vi "Create chapter and section.vi"(0 "PDF Report IN":refnum<class "PDF Report Class.lvclass">, 2 "TriggerNewPage":bool, 5 "Chapter or section IN":T1, 7 "Paragragh":refnum<k24>, 11 "error in (no error)":errorcluster, 13 "BookmarkOpen":bool=TRUE) -> (4 "PDF Report OUT":refnum<class "PDF Report Class.lvclass">, 8 "Chapter":refnum<k24>, 10 "Section":refnum<k24>, 15 "error out":errorcluster)   [LabVIEW 2019]
doc: "Version 1.1\nDeveloped by Jean-Marc Simard\nCopyright © 2012, Exaprom Inc.\nAll rights reserved.\nLicense: BSD\n\nWith iTextSharp 4.1.6 (http://itextsharp.sourceforge.net)\nunder Mozilla Public License Version 1.1\n(http://www.mozilla.org/MPL/MPL-1.1.html)"
uses:
  <userlib>/Exaprom PDF/LV Class/PDF Report Class/PDF Report Class.lvclass
  <userlib>/Exaprom PDF/Controls/Chapter Controls/Chapter.ctl
  C:/Program Files/National Instruments/LabVIEW 2019/user.lib/Exaprom PDF/DLL/itextsharp.dll
  DLL/itextsharp.dll
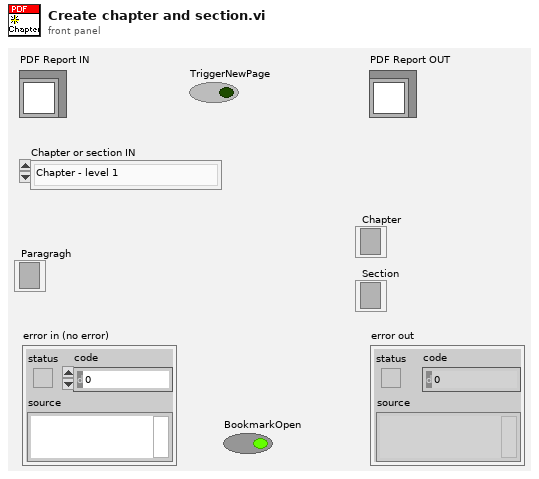
[diagram p1: front panel]
types:
  T1 = typedef "Chapter.ctl" = enum16{"Chapter - level 1", "Chapter - level 2", "Chapter - level 3", "Chapter - level 4"}
  T2 = cluster{"ChapterAutoNumber":refnum<k24>, "Section [ ]":refnum<k24>[]}
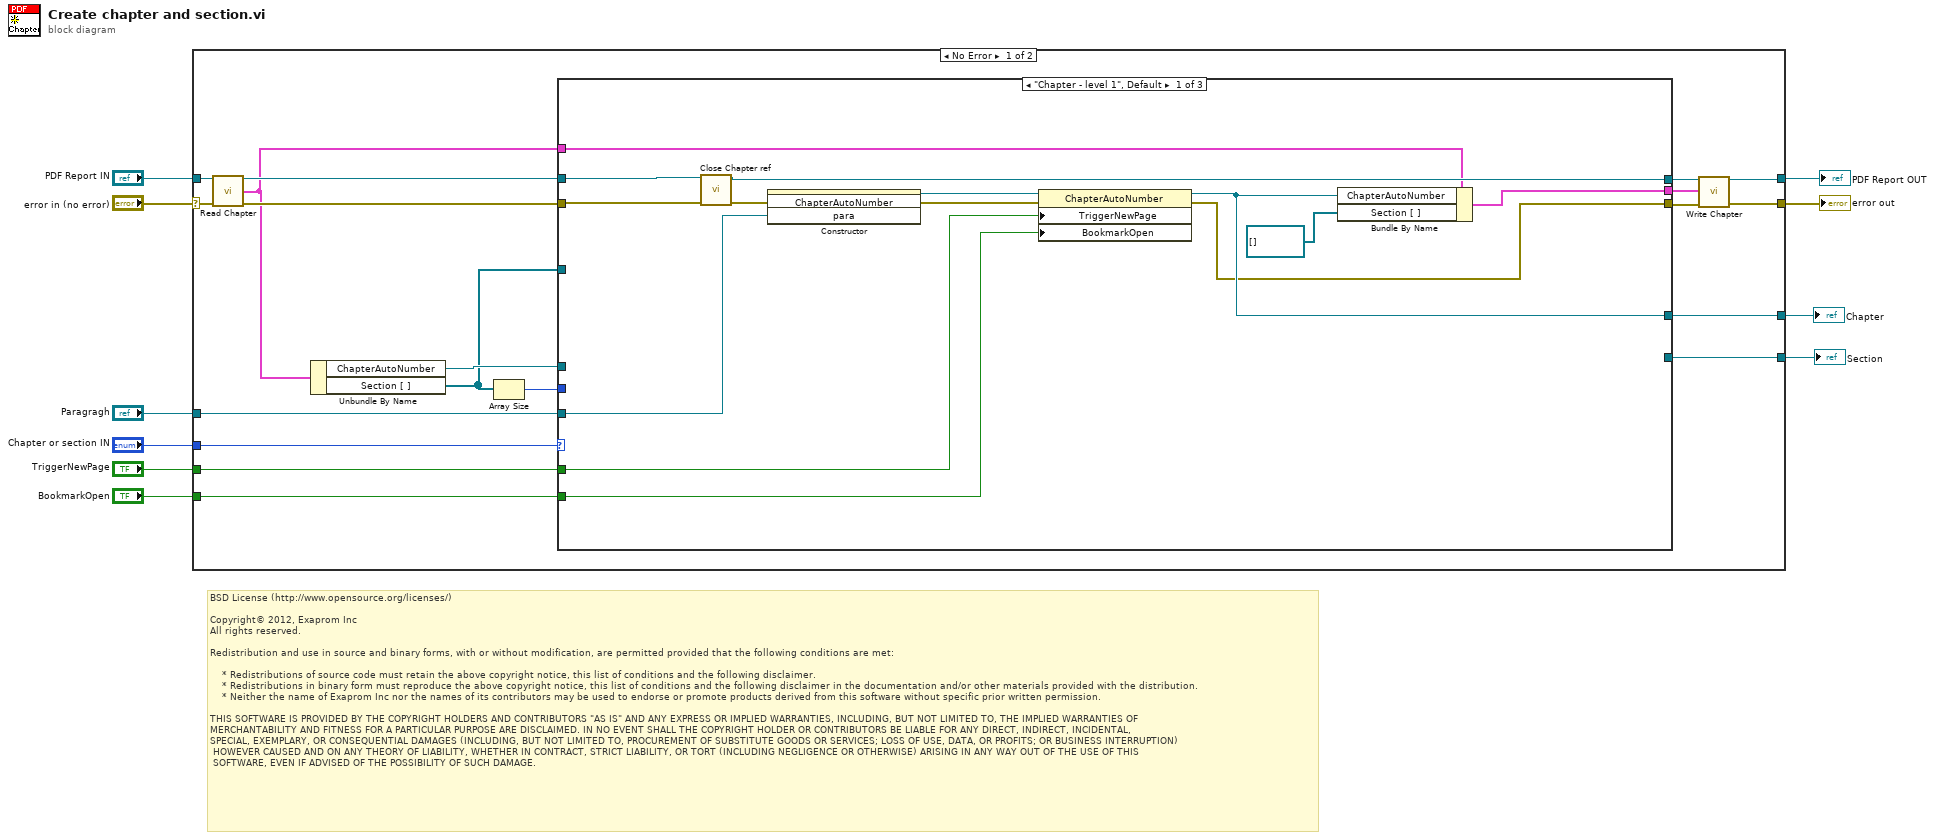
[diagram p0: block diagram]
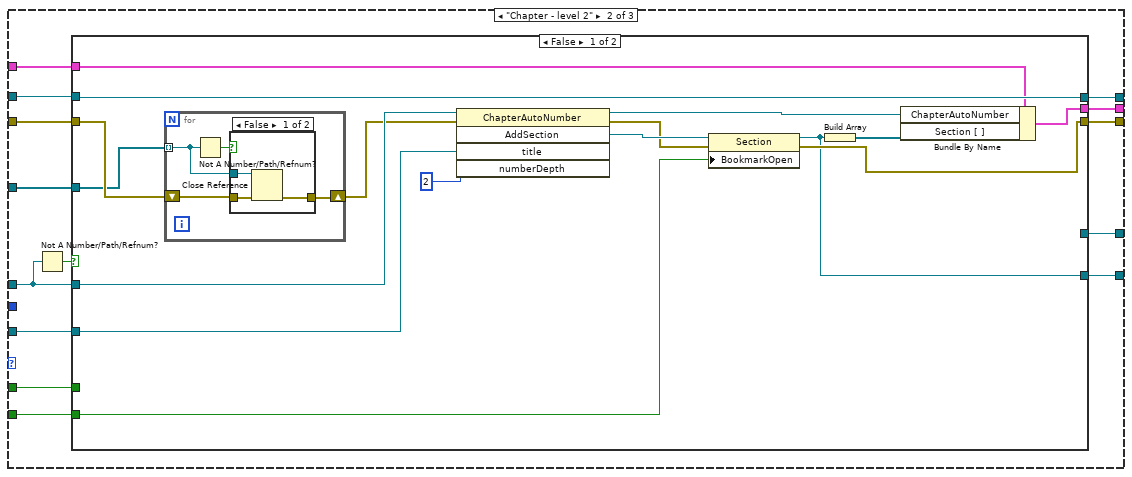
[diagram p2: hidden frame]
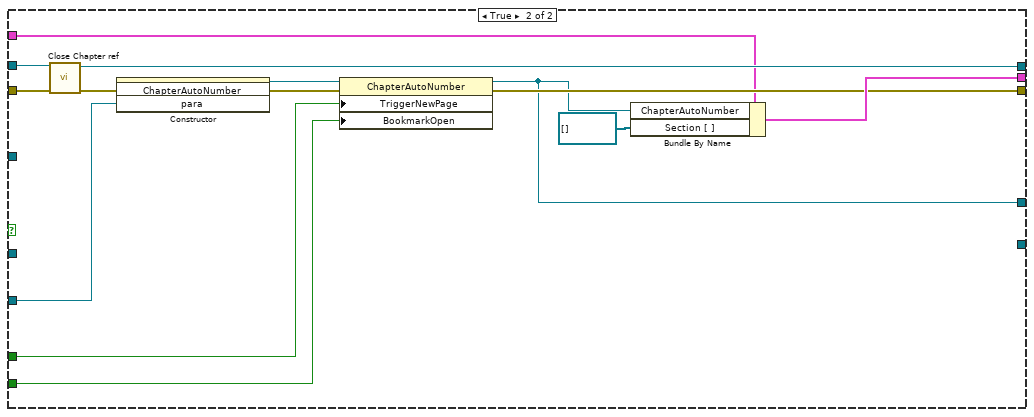
[diagram p4: hidden frame]
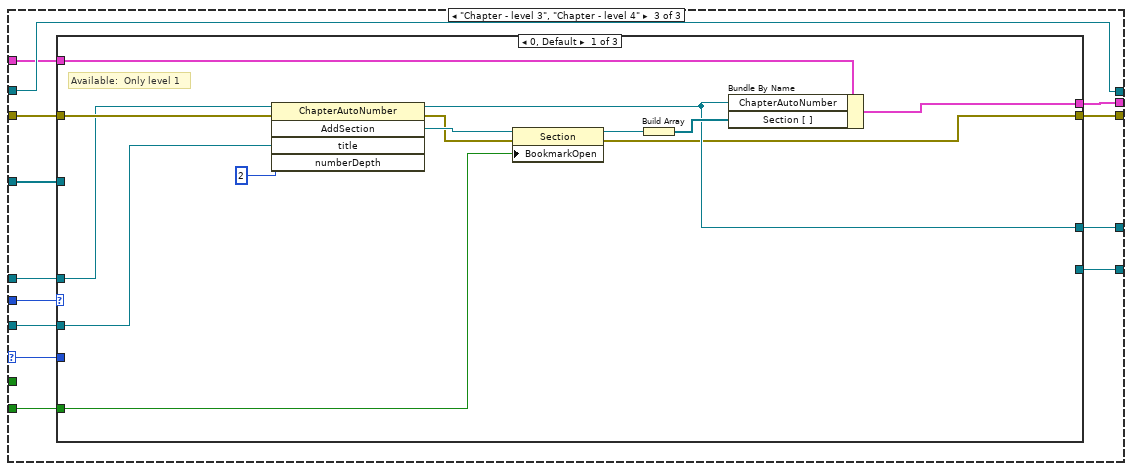
[diagram p5: hidden frame]
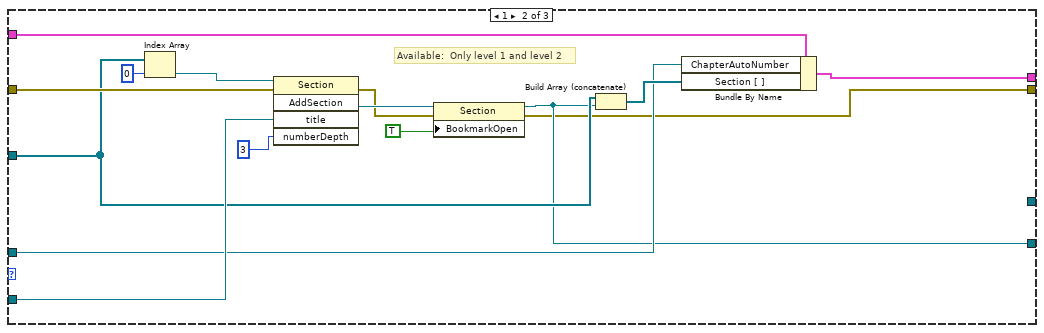
[diagram p6: hidden frame]
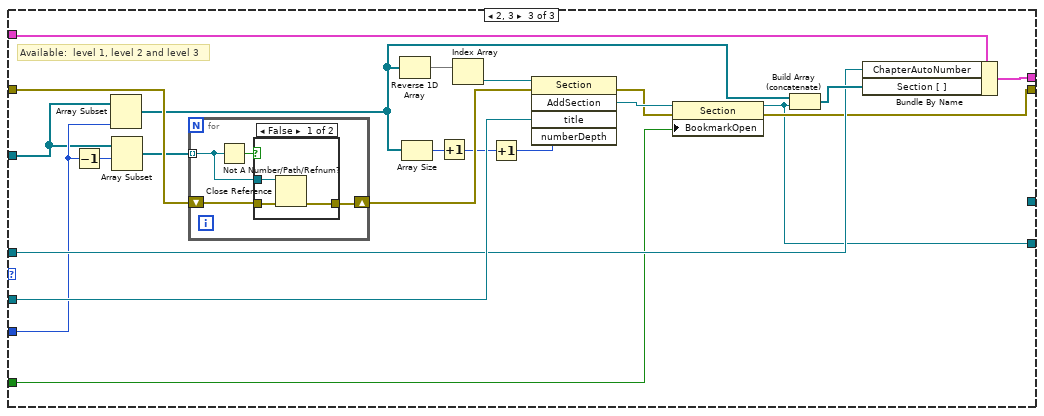
[diagram p7: hidden frame]
diagram:
  # "BSD License (http://www.opensource.org/licenses/)\n\nCopyright© 2012, Exaprom Inc\nAll rights reserved.\n\nRedistribution and use in source and binary forms, with or without modification, are permitted provided that the following conditions are met:\n\n    * Redistributions of source code must retain the above copyright notice, this list of conditions and the following disclaimer.\n    * Redistributions in binary form must reproduce the above copyright notice, this list of conditions and the following disclaimer in the documentation and/or other materials provided with the distribution.\n    * Neither the name of Exaprom Inc nor the names of its contributors may be used to endorse or promote products derived from this software without specific prior written permission.\n\nTHIS SOFTWARE IS PROVIDED BY THE COPYRIGHT HOLDERS AND CONTRIBUTORS \"AS IS\" AND ANY EXPRESS OR IMPLIED WARRANTIES, INCLUDING, BUT NOT LIMITED TO, THE IMPLIED WARRANTIES OF \nMERCHANTABILITY AND FITNESS FOR A PARTICULAR PURPOSE ARE DISCLAIMED. IN NO EVENT SHALL THE COPYRIGHT HOLDER OR CONTRIBUTORS BE LIABLE FOR ANY DIRECT, INDIRECT, INCIDENTAL,\nSPECIAL, EXEMPLARY, OR CONSEQUENTIAL DAMAGES (INCLUDING, BUT NOT LIMITED TO, PROCUREMENT OF SUBSTITUTE GOODS OR SERVICES; LOSS OF USE, DATA, OR PROFITS; OR BUSINESS INTERRUPTION)\n HOWEVER CAUSED AND ON ANY THEORY OF LIABILITY, WHETHER IN CONTRACT, STRICT LIABILITY, OR TORT (INCLUDING NEGLIGENCE OR OTHERWISE) ARISING IN ANY WAY OUT OF THE USE OF THIS\n SOFTWARE, EVEN IF ADVISED OF THE POSSIBILITY OF SUCH DAMAGE."
  n1 = case shown="No Error" "error in (no error)" {
    selector: "error in (no error)" -> [w28 w168]
    tunnel: "PDF Report IN" -> [w29 w167]
    tunnel: [w18 w167] -> w9
    tunnel: [w21 w168] -> w8
    tunnel: "Chapter or section IN" -> [w27 _]
    tunnel: "Paragragh" -> [w23 _]
    tunnel: [w15 _] -> w4
    tunnel: [w14 _] -> w3
    tunnel: "TriggerNewPage" -> [w13 _]
    tunnel: "BookmarkOpen" -> [w11 _]
    frame No Error {
      n2 = call-dynamic "Read Chapter.vi"("PDF Report Class in"=w29, "error in (no error)"=w28) -> ("PDF Report Class out"=w17:refnum<class "PDF Report Class.lvclass">, "Chapter ref"=w12:T2, "error out"=w26:errorcluster)  [unwired: 11 in]
      n3 = Unbundle By Name(w12) -> ("ChapterAutoNumber"=w24:refnum<k24>, "Section [ ]"=w22:refnum<k24>[])
      n4 = Array Size(array=w22) -> (size(s)=w25:i32)
      n5 = case shown="\"Chapter - level 1\", Default" w27 {
        selector: w27 -> [_ _ w101]
        tunnel: w26 -> [w34 w56 w104]
        tunnel: w25 -> [_ _ w108]
        tunnel: w24 -> [_ w51 w103]
        tunnel: w23 -> [w36 w57 w102]
        tunnel: [w32 w53 w105] -> w20
        tunnel: w22 -> [_ w55 w107]
        tunnel: [w39 w54 w106] -> w19
        tunnel: w17 -> [w33 w50 w100]
        tunnel: [w41 w49 w100] -> w16
        tunnel: [w37 w48 w98] -> w15
        tunnel: [_ w47 w99] -> w14
        tunnel: w13 -> [w38 w46 _]
        tunnel: w12 -> [w35 w45 w97]
        tunnel: w11 -> [w31 w44 w96]
        frame "Chapter - level 1", Default {
          n6 = call <userlib>:"Close Chapter ref.vi"("PDF Report IN"=w33, "error in (no error)"=w34) -> ("PDF Report OUT"=w41:refnum<class "PDF Report Class.lvclass">, "error out"=w42:errorcluster)  [unwired: 12 in]
          n7 = constructor class="ChapterAutoNumber"(error in=w42, "para"=w36) -> (reference out=w30:refnum<k24>, error out=w43:errorcluster)  [unwired: 2 in, 2 out]
          n8 = property class="ChapterAutoNumber"(reference=w30, error in=w43, "TriggerNewPage"=w38, "BookmarkOpen"=w31) -> (reference out=w37:refnum<k24>, error out=w32:errorcluster)
          n9 = Bundle By Name(cluster=w35, "ChapterAutoNumber"=w37, "Section [ ]"=refnum<k24>[] []) -> (w39:T2)
        }
        frame "Chapter - level 2" {
          n10 = Not A Number/Path/Refnum?(number/path/refnum=w51) -> (NaN/Path/Refnum?=w52:bool)
          n11 = case shown="False" w52 {
            tunnel: w51 -> [w73 _]
            tunnel: w57 -> [w72 w86]
            tunnel: w56 -> [w68 w91]
            tunnel: w55 -> [w66 _]
            tunnel: [w65 w90] -> w54
            tunnel: [w62 w88] -> w53
            tunnel: w50 -> [w61 w89]
            tunnel: [w61 w87] -> w49
            tunnel: [_ w85] -> w48
            tunnel: [w60 _] -> w47
            tunnel: w46 -> [_ w83]
            tunnel: w45 -> [w59 w84]
            tunnel: w44 -> [w58 w82]
            frame False {
              n12 = for {
                shift-right: [w75] -> w67
                shift-left: w68 -> [w76]
                tunnel: w66 -> [w74] mode=indexing
                n13 = Not A Number/Path/Refnum?(number/path/refnum=w74) -> (NaN/Path/Refnum?=w77:bool)
                n14 = case shown="False" w77 {
                  tunnel: w74 -> [w80 _]
                  tunnel: w76 -> [w79 w81]
                  tunnel: [w78 w81] -> w75
                  frame False {
                    n15 = Close Reference(reference=w80, error in (no error)=w79) -> (error out=w78:errorcluster)
                  }
                  frame True {
                  }
                }
              }
              n16 = invoke class="ChapterAutoNumber" method="AddSection"(reference=w73, error in=w67, "title"=w72, "numberDepth"=2) -> (reference out=w69:refnum<k24>, error out=w63:errorcluster, "AddSection"=w64:refnum<k24>)  [unwired: 1 in, 2 out]
              n17 = property class="Section"(reference=w64, error in=w63, "BookmarkOpen"=w58) -> (reference out=w60:refnum<k24>, error out=w62:errorcluster)
              n18 = Build Array(w60) -> (w70:refnum<k24>[])
              n19 = Bundle By Name(cluster=w59, "ChapterAutoNumber"=w69, "Section [ ]"=w70) -> (w65:T2)
            }
            frame True {
              n20 = call <userlib>:"Close Chapter ref.vi"("PDF Report IN"=w89, "error in (no error)"=w91) -> ("PDF Report OUT"=w87:refnum<class "PDF Report Class.lvclass">, "error out"=w93:errorcluster)  [unwired: 12 in]
              n21 = constructor class="ChapterAutoNumber"(error in=w93, "para"=w86) -> (reference out=w94:refnum<k24>, error out=w95:errorcluster)  [unwired: 2 in, 2 out]
              n22 = property class="ChapterAutoNumber"(reference=w94, error in=w95, "TriggerNewPage"=w83, "BookmarkOpen"=w82) -> (reference out=w85:refnum<k24>, error out=w88:errorcluster)
              n23 = Bundle By Name(cluster=w84, "ChapterAutoNumber"=w85, "Section [ ]"=refnum<k24>[] []) -> (w90:T2)
            }
          }
        }
        frame "Chapter - level 3", "Chapter - level 4" {
          n24 = case shown="0, Default" w108 {
            tunnel: w107 -> [_ w128 w148]
            tunnel: [w112 w123 w142] -> w105
            tunnel: [w119 w134 w156] -> w106
            tunnel: w104 -> [w118 w133 w158]
            tunnel: w103 -> [w117 w129 w154]
            tunnel: w102 -> [w111 w132 w155]
            tunnel: w101 -> [_ _ w151]
            tunnel: [_ w124 w141] -> w99
            tunnel: [w116 _ _] -> w98
            tunnel: w97 -> [w110 w122 w138]
            tunnel: w96 -> [w109 _ w137]
            frame 0, Default {
              # "Available:  Only level 1"
              n25 = invoke class="ChapterAutoNumber" method="AddSection"(reference=w117, error in=w118, "title"=w111, "numberDepth"=2) -> (reference out=w116:refnum<k24>, error out=w113:errorcluster, "AddSection"=w114:refnum<k24>)  [unwired: 1 in, 2 out]
              n26 = property class="Section"(reference=w114, error in=w113, "BookmarkOpen"=w109) -> (reference out=w115:refnum<k24>, error out=w112:errorcluster)
              n27 = Build Array(w115) -> (w120:refnum<k24>[])
              n28 = Bundle By Name(cluster=w110, "ChapterAutoNumber"=w116, "Section [ ]"=w120) -> (w119:T2)
            }
            frame 1 {
              # "Available:  Only level 1 and level 2"
              n29 = Index Array(array=w128, index=0) -> (element=w130:refnum<k24>)
              n30 = invoke class="Section" method="AddSection"(reference=w130, error in=w133, "title"=w132, "numberDepth"=3) -> (error out=w125:errorcluster, "AddSection"=w126:refnum<k24>)  [unwired: 1 in, 3 out]
              n31 = property class="Section"(reference=w126, error in=w125, "BookmarkOpen"=TRUE) -> (reference out=w124:refnum<k24>, error out=w123:errorcluster)
              n32 = Build Array (concatenate)(w128, w124) -> (w135:refnum<k24>[])
              n33 = Bundle By Name(cluster=w122, "ChapterAutoNumber"=w129, "Section [ ]"=w135) -> (w134:T2)
            }
            frame 2, 3 {
              # "Available:  level 1, level 2 and level 3"
              n34 = Decrement(x=w151) -> (x-1=w153:T1)
              n35 = Array Subset(array=w148, length=w151) -> (w146:refnum<k24>[])  [unwired: 1 in]
              n36 = Array Subset(array=w148, index=w153) -> (w152:refnum<k24>[])  [unwired: 1 in]
              n37 = for {
                shift-right: [w160] -> w147
                shift-left: w158 -> [w161]
                tunnel: w152 -> [w159] mode=indexing
                n38 = Not A Number/Path/Refnum?(number/path/refnum=w159) -> (NaN/Path/Refnum?=w162:bool)
                n39 = case shown="False" w162 {
                  tunnel: w159 -> [w165 _]
                  tunnel: w161 -> [w164 w166]
                  tunnel: [w163 w166] -> w160
                  frame False {
                    n40 = Close Reference(reference=w165, error in (no error)=w164) -> (error out=w163:errorcluster)
                  }
                  frame True {
                  }
                }
              }
              n41 = Reverse 1D Array(array=w146) -> (reversed array=w150:refnum<k24>[])
              n42 = Array Size(array=w146) -> (size(s)=w145:i32)
              n43 = Increment(x=w145) -> (x+1=w140:i32)
              n44 = Index Array(array=w150) -> (element=w149:refnum<k24>)  [unwired: 1 in]
              n45 = Increment(x=w140) -> (x+1=w139:i32)
              n46 = invoke class="Section" method="AddSection"(reference=w149, error in=w147, "title"=w155, "numberDepth"=w139) -> (error out=w143:errorcluster, "AddSection"=w144:refnum<k24>)  [unwired: 1 in, 3 out]
              n47 = property class="Section"(reference=w144, error in=w143, "BookmarkOpen"=w137) -> (reference out=w141:refnum<k24>, error out=w142:errorcluster)
              n48 = Build Array (concatenate)(w146, w141) -> (w157:refnum<k24>[])
              n49 = Bundle By Name(cluster=w138, "ChapterAutoNumber"=w154, "Section [ ]"=w157) -> (w156:T2)
            }
          }
        }
      }
      n50 = call-dynamic "Write Chapter.vi"("PDF Report Class in"=w16, "Chapter ref"=w19, "error in (no error)"=w20) -> ("PDF Report Class out"=w18:refnum<class "PDF Report Class.lvclass">, "error out"=w21:errorcluster)  [unwired: 11 in]
    }
    frame Error {
    }
  }
  "PDF Report OUT" <- w9
  "error out" <- w8
  "Chapter" <- w4
  "Section" <- w3
